vi "NATS CLOSE.vi"(8 "error in":errorcluster, 11 "nats connection in":T1={"connection ID"=refnum, "server INFO"="", "timeout ms"=5000, "verbose?"=FALSE, "server headers?"=FALSE, "client headers?"=FALSE}) -> (0 "error out":errorcluster)   [LabVIEW 2013, in "NATS Core.lvlib"]
doc: "Closes the TCP connection to the NATS server."
uses:
  NATS Core.lvlib
  Controls/nats connection.ctl
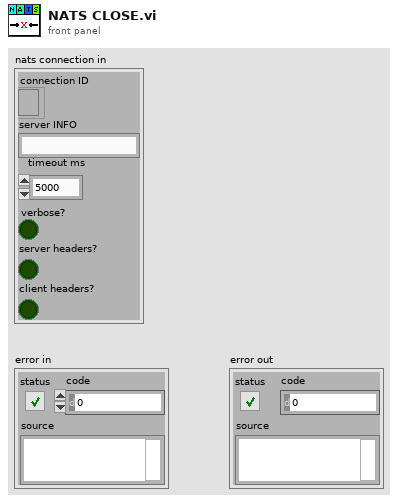
[diagram p1: front panel]
types:
  T1 = typedef "NATS Core.lvlib/nats connection.ctl" = cluster{"connection ID":refnum<k5>, "server INFO":string, "timeout ms":i32, "verbose?":bool, "server headers?":bool, "client headers?":bool}
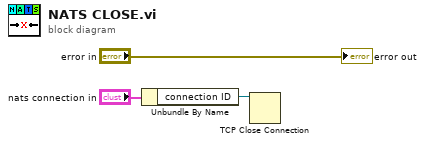
[diagram p0: block diagram]
diagram:
  n1 = Unbundle By Name("nats connection in") -> ("connection ID"=w3:refnum<k5>)
  n2 = TCP Close Connection(connection ID=w3) -> ()  [unwired: 2 in, 2 out]
  "error out" <- "error in"
